vi "Prepare Get Joystick State Msg.vi"(8 "error in (no error)":errorcluster, 11 "RPI.SenseHat.Actor in":refnum<class "RPI.SenseHat.Actor.lvclass">) -> (0 "error out":errorcluster, 3 "RPI.SenseHat.Actor out":refnum<class "RPI.SenseHat.Actor.lvclass">)   [LabVIEW 2020, in "RPI.SenseHat.Actor.lvlib" / "RPI.SenseHat.Actor.lvclass"]
uses:
  RPI.SenseHat.Actor.lvclass
  C:/Program Files (x86)/National Instruments/LabVIEW 2020/vi.lib/ActorFramework/Actor/Actor.lvclass
  RPI.SenseHat.Actor Messages/Get Joystick State Msg/Update Joystick State Msg.lvclass
  C:/Program Files (x86)/National Instruments/LabVIEW 2020/vi.lib/ActorFramework/Message/Message.lvclass
  <vilib>/ActorFramework/Actor/Actor.lvclass/Actor.ctl
  <vilib>/ActorFramework/Message Enqueuer/Message Enqueuer.lvclass/Message Enqueuer.ctl
  RPI.SenseHat.Actor.lvclass/RPI.SenseHat.Actor.ctl
  <vilib>/ActorFramework/Message Enqueuer/Init from Existing Queue.vi
  <vilib>/ActorFramework/Message Enqueuer/Message Enqueuer.lvclass
  <vilib>/ActorFramework/Actor/Actor.lvclass
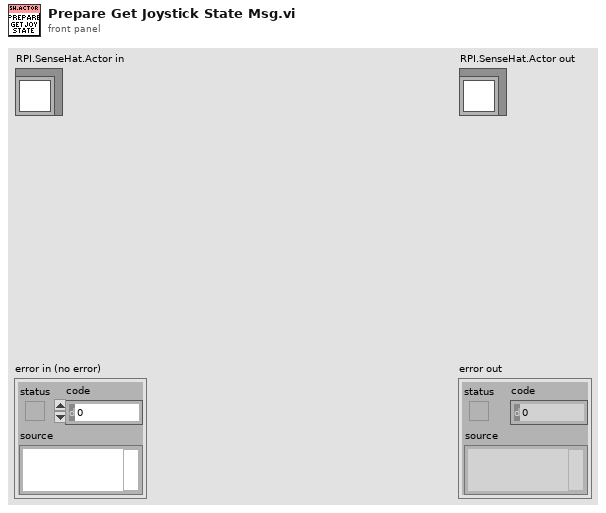
[diagram p1: front panel]
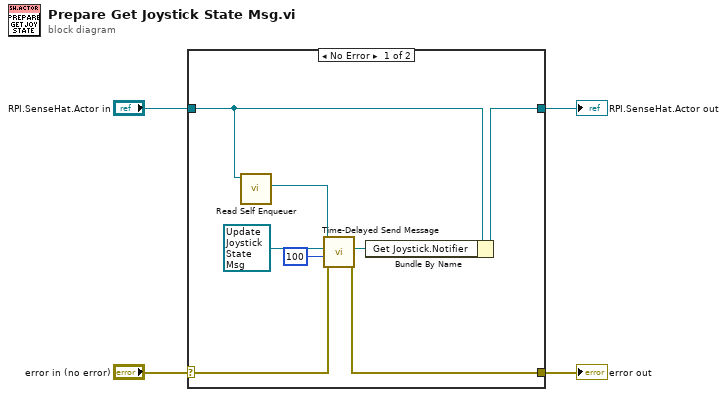
[diagram p0: block diagram]
diagram:
  n1 = case shown="No Error" "error in (no error)" {
    selector: "error in (no error)" -> [w6 w14]
    tunnel: [w5 w14] -> w3
    tunnel: [w8 w13] -> w1
    tunnel: "RPI.SenseHat.Actor in" -> [w10 w13]
    frame No Error {
      n2 = call <vilib>:"Read Self Enqueuer.vi"("Actor"=w10) -> ("Self Enqueuer"=w9:refnum<class "Message Enqueuer.lvclass">)  [unwired: 10 in]
      n3 = call <vilib>:"Time-Delayed Send Message.vi"("error in (no error)"=w6, "Milliseconds To Wait"=100, "Message"=refnum<class "Update Joystick State Msg.lvclass"> refnum ("RPI.SenseHat.Actor.lvlib:Get Joystick State Msg.lvclass"), "Message Enqueuer"=w9) -> ("error out"=w5:errorcluster, "Delivery Notifier"=w7:refnum<notifier>)  [unwired: 6 in]
      n4 = Bundle By Name(cluster=w10, "Get Joystick.Notifier"=w7) -> (w8:refnum<class "RPI.SenseHat.Actor.lvclass">)
    }
    frame Error {
    }
  }
  "error out" <- w3
  "RPI.SenseHat.Actor out" <- w1
